vi "test.vi"() -> ()   [LabVIEW 2020, in "GraphBG_manage.lvlib" / "Graph.lvclass"]
uses:
  Graph.lvclass
  T50/subVI/xyY_graph.ctl
panel:
  out "error out":errorcluster
  in  "stop":bool
  out "xyY_Graph":T1
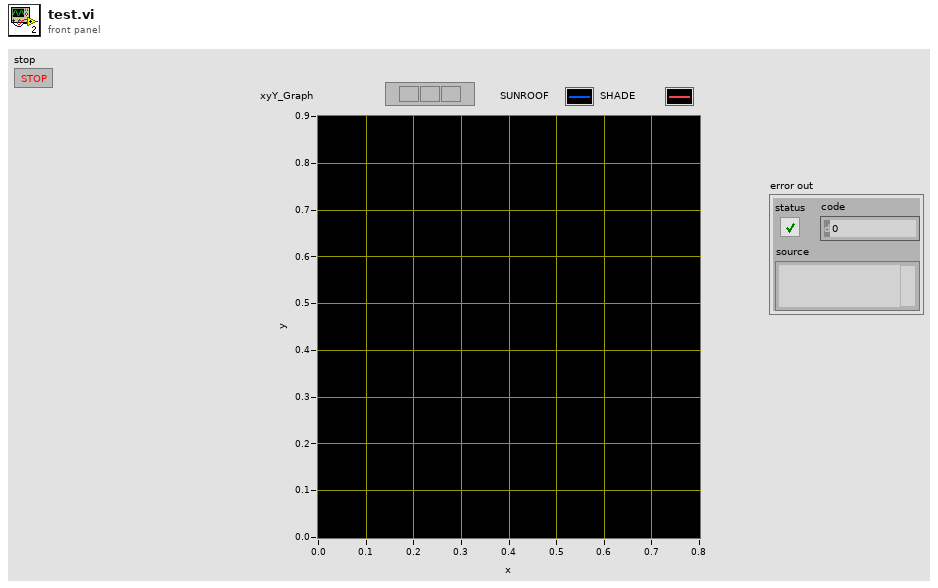
[diagram p1: front panel]
types:
  T1 = typedef "xyY_graph.ctl" = cluster{"Y":dbl[], "Y":dbl[]}[]
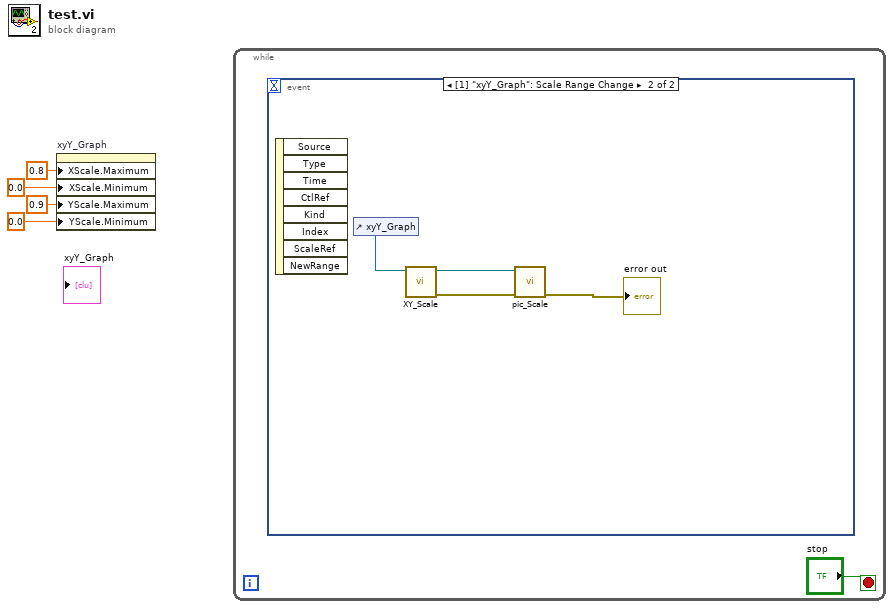
[diagram p0: block diagram]
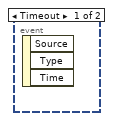
[diagram p2: hidden frame]
diagram:
  n1 = property on="xyY_Graph" class="XYGraph (strict)"("XScale.Maximum"=0.8 ("X Scale.Range:Maximum"), "XScale.Minimum"=0.0 ("X Scale.Range:Minimum"), "YScale.Maximum"=0.9 ("Y Scale.Range:Maximum"), "YScale.Minimum"=0.0 ("Y Scale.Range:Minimum")) -> ()  [unwired: 2 in, 2 out]
  n2 = while {
    stop <- "stop" stop-if-true
    n3 = event shown="[1] \"xyY_Graph\": Scale Range Change" {
      selector: _ -> [_ _]
      dyn-events: _ -> [_ _]
      timeout: _ -> [_ _]
      event Timeout {
        n4 = event-data() -> ()  [unwired: 1 in, 3 out]
      }
      event Scale Range Change {
        n5 = event-data() -> ()  [unwired: 1 in, 8 out]
        n6 = control-ref of="xyY_Graph"() -> (w9:refnum<vi>)
        n7 = call "XY_Scale.vi"("Graph_ref_in"=w9) -> ("error out"=w8:errorcluster, "Graph_ref_out"=w7:refnum<vi>)  [unwired: 9 in]
        n8 = call "pic_Scale.vi"("error in (no error)"=w8, "Graph_ref_in"=w7) -> ("error out"=→"error out":errorcluster)  [unwired: 8 in, 1 out]
      }
    }
  }
